vi "Stopping.vi"(6 "Teller":T1 {"AbsoluteTime" format="%<%x %.3X>T"}, 8 "Error in":errorcluster, 11 "Base Actor in":refnum<class "BaseActor.lvclass">) -> (0 "Error out":errorcluster, 3 "Base Actor out":refnum<class "BaseActor.lvclass">)   [LabVIEW 2020, in "jettl.lvlib" / "BaseActor.lvlib" / "BaseActor.lvclass"]
doc: "jettl 6.12.1.94\nNathan Davis - Nathan Davis\nCopyright (c) 2026, Nathan Davis\nMIT"
uses:
  BaseActor.lvclass
  BaseActor.lvclass/BaseActor.ctl
  jettl.lvlib
  MessageMetadata.ctl
  Lifetime.ctl
  TellOrigin.ctl
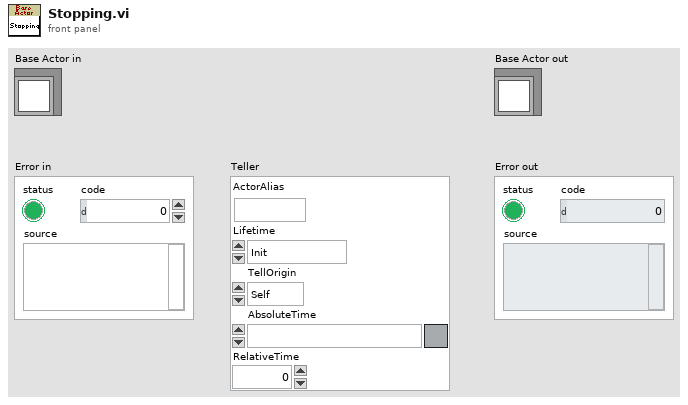
[diagram p1: front panel]
types:
  T1 = typedef "jettl.lvlib/MessageMetadata.ctl" = cluster{"ActorAlias":string, "Lifetime":T2, "TellOrigin":T3, "AbsoluteTime":timestamp, "RelativeTime":dbl}
  T2 = typedef "jettl.lvlib/Lifetime.ctl" = enum16{"Init", "Spawn", "Setup", "TeardownBeforeRunning", "Running", "StopCalled", "StoppingWithComponents", "StoppingNoComponents", "TeardownAfterRunning", "Stopped"}
  T3 = typedef "jettl.lvlib/TellOrigin.ctl" = enum16{"Self", "Mediator", "Component"}
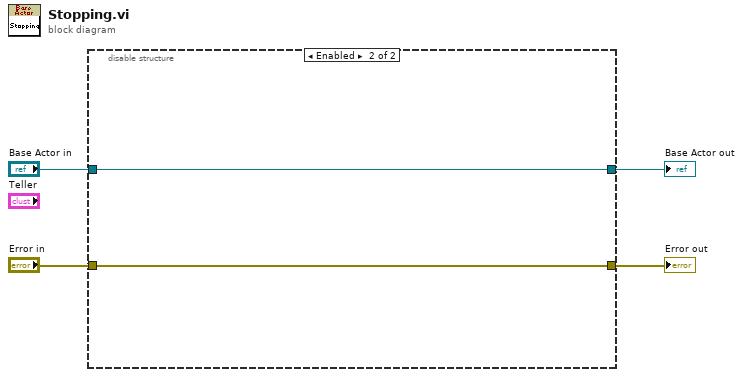
[diagram p0: block diagram]
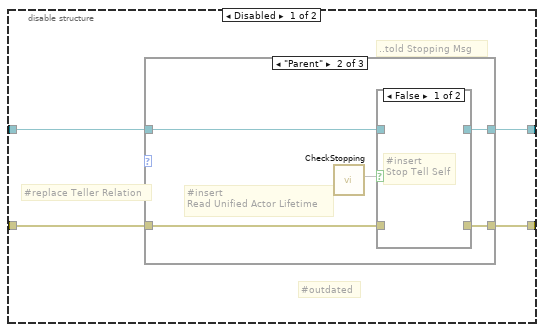
[diagram p2: hidden frame]
diagram:
  n1 = disable-structure shown="Enabled" {
    disable-tunnel: "Base Actor in" -> [w8 w25]
    disable-tunnel: [w7 w25] -> w3
    disable-tunnel: "Error in" -> [w6 w24]
    disable-tunnel: [w5 w24] -> w1
    frame Disabled {
      # "#outdated"
      # "#replace Teller Relation"
      # "..told Stopping Msg"
      n2 = case shown="\"Parent\"" {
        selector: _ -> [_ _ _]
        tunnel: w8 -> [w10 w12 w23]
        tunnel: [w10 w16 w23] -> w7
        tunnel: w6 -> [w9 w15 w22]
        tunnel: [w9 w14 w22] -> w5
        frame "Self" {
          # "Case will not fundamentally execute"
        }
        frame "Parent" {
          # "#insert\nRead Unified Actor Lifetime"
          n3 = call "CheckStopping.vi"() -> (2:w13, 10:w11)  [unwired: 9 in, 1 out]
          n4 = case shown="False" w13 {
            tunnel: [w19 w21] -> w16
            tunnel: w15 -> [w18 w20]
            tunnel: [_ w20] -> w14
            tunnel: w12 -> [w17 w21]
            frame False {
              # "#insert\nStop Tell Self"
            }
            frame True {
            }
          }
        }
        frame "Child" {
          # "Case will not fundamentally execute"
        }
      }
    }
    frame Enabled {
    }
  }
  "Base Actor out" <- w3
  "Error out" <- w1
